vi "create scan vectr2.1.vi"(3 "Table Control":string[][](table)) -> (0 "parameters":dbl[](array[numeric]), 2 "positions":dbl[](array[numeric]))   [LabVIEW 2020]
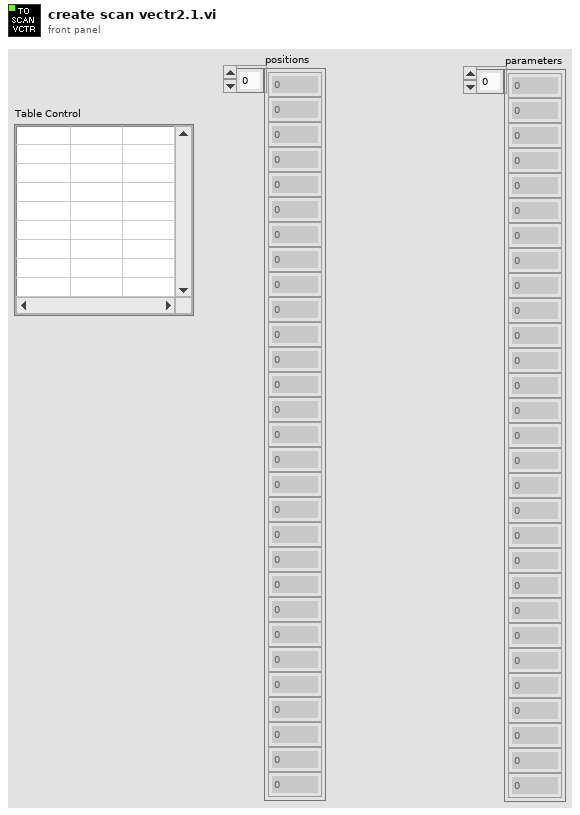
[diagram p1: front panel]
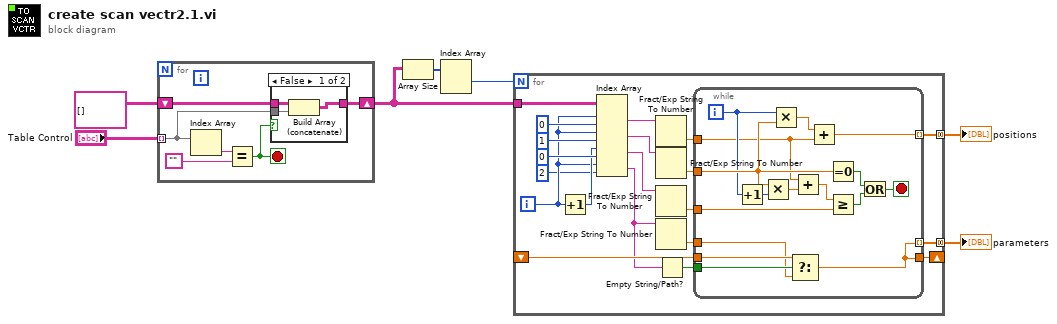
[diagram p0: block diagram]
diagram:
  n1 = for {
    tunnel: "Table Control" -> [w9] mode=indexing
    shift-right: [w8] -> w4
    shift-left: string[][] [] ("t") -> [w11]
    stop <- w10 stop-if-true
    n2 = Index Array(array=w9) -> (element=w12:string)  [unwired: 1 in]
    n3 = Equal?(x=w12, y="") -> (x = y?=w10:bool)
    n4 = case shown="False" w10 {
      tunnel: w11 -> [w16 w17]
      tunnel: w9 -> [w15 _]
      tunnel: [w14 w17] -> w8
      frame False {
        n5 = Build Array (concatenate)(w16, w15) -> (w14:string[][])
      }
      frame True {
      }
    }
  }
  n6 = Array Size(array=w4) -> (size(s)=w3:i32[])
  n7 = Index Array(array=w3) -> (element #1=w2:i32)  [unwired: 2 in, 1 out]
  n8 = for {
    N: w2 -> [_]
    tunnel: w4 -> [w33]
    tunnel: [w26] -> w5 mode=concatenating
    tunnel: [w22] -> w1 mode=concatenating
    shift-right: [w21] -> _
    shift-left: _ -> [w20]
    i -> [w25]
    n9 = Increment(x=w25) -> (x+1=w35:i32)
    n10 = Index Array(array=w33, index (row) #1=w25, index (col) #1=0 ("disabled index (col)"), index (row) #2=w25, index (col) #2=1 ("disabled index (col)"), index (row) #3=w35, index (col) #3=0 ("disabled index (col)"), index (row) #4=w25, index (col) #4=2 ("disabled index (col)")) -> (element #1=w32:string, element #2=w31:string, element #3=w30:string, element #4=w19:string)
    n11 = Fract/Exp String To Number(string=w32) -> (number=w29:dbl)  [unwired: 3 in, 1 out]
    n12 = Fract/Exp String To Number(string=w31) -> (number=w28:dbl)  [unwired: 3 in, 1 out]
    n13 = Fract/Exp String To Number(string=w30) -> (number=w27:dbl)  [unwired: 3 in, 1 out]
    n14 = Fract/Exp String To Number(string=w19) -> (number=w23:dbl)  [unwired: 3 in, 1 out]
    n15 = Empty String/Path?(string/path=w19) -> (empty?=w18:bool)
    n16 = while {
      tunnel: w29 -> [w43]
      tunnel: w28 -> [w45]
      tunnel: w27 -> [w49]
      tunnel: [w53] -> w26 mode=indexing
      tunnel: w23 -> [w39]
      tunnel: [w38] -> w22 mode=indexing
      tunnel: [w38] -> w21
      tunnel: w20 -> [w40]
      tunnel: w18 -> [w41]
      i -> [w44]
      stop <- w46 stop-if-true
      n17 = Increment(x=w44) -> (x+1=w51:i32)
      n18 = Multiply(x=w45, y=w51) -> (x*y=w52:dbl)
      n19 = Multiply(x=w44, y=w45) -> (x*y=w42:dbl)
      n20 = Select(t=w40, s=w41, f=w39) -> (s? t:f=w38:dbl)
      n21 = Add(x=w43, y=w52) -> (x+y=w50:dbl)
      n22 = Add(x=w42, y=w43) -> (x+y=w53:dbl)
      n23 = Equal To 0?(x=w45) -> (x = 0?=w48:bool)
      n24 = Greater Or Equal?(x=w50, y=w49) -> (x >= y?=w47:bool)
      n25 = Or(x=w48, y=w47) -> (x .or. y?=w46:bool)
    }
  }
  "positions" <- w5
  "parameters" <- w1
